vi "Wait For Single Object.vi"(8 "error in":errorcluster, 10 "Timeout":u32=4294967295 format="%d ms", 11 "Read Event in":refnum<class "Read Event.lvclass">) -> (0 "error out":errorcluster, 2 "Timed Out":bool, 3 "Read Event out":refnum<class "Read Event.lvclass">)   [LabVIEW 2019, in "PCANBasic.lvlib" / "Read Event.lvclass"]
doc: "Waits until the specified object is in the signaled state or the time-out interval elapses.\n\nThe time-out interval, in milliseconds. If a nonzero value is specified, the function waits until the object is signaled or the interval elapses. If dwMilliseconds is zero, the function does not enter a wait state if the object is not signaled; it always returns immediately. If dwMilliseconds is INFINITE (0xFFFFFFFF), the function will return only when the object is signaled."
uses:
  Read Event.lvclass
  Read Event.lvclass/Read Event.ctl
  PCANBasic.lvlib
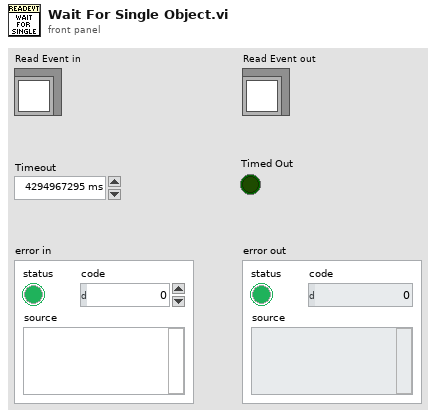
[diagram p1: front panel]
types:
  T1 = typedef "PCANBasic.lvlib/Read Event.lvclass/Event Handle.ctl" = u64
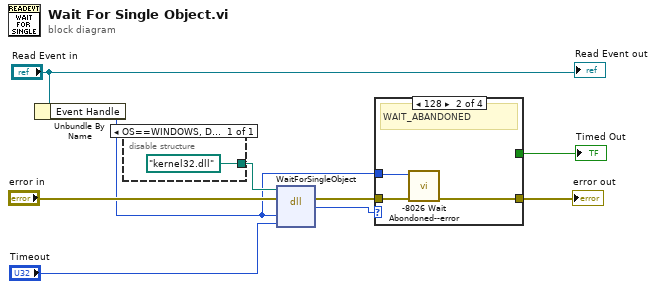
[diagram p0: block diagram]
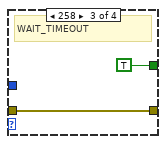
[diagram p3: hidden frame]
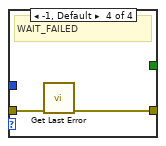
[diagram p4: hidden frame]
diagram:
  n1 = Unbundle By Name("Read Event in") -> ("Event Handle"=w2:T1)
  n2 = disable-structure shown="OS==WINDOWS, Default" {
    disable-tunnel: [path "kernel32.dll" ("path in")] -> w9
    frame condition #0 (active) {
    }
  }
  n3 = dll-call lib="?" fn="WaitForSingleObject"(path in=w9, error in="error in", "hdlEvent"=w2, "Timeout"="Timeout") -> (error out=w6:errorcluster, "result"=w5:u32)  [unwired: 3 in, 1 out]
  n4 = case "success?" shown="128" w5 {
    tunnel: w6 -> [w11 w14 w16 w18]
    tunnel: [w11 w13 w16 w17] -> w4
    tunnel: [_ _ TRUE _] -> w3
    tunnel: w2 -> [_ w12 _ _]
    frame 0 {
      # "WAIT_OBJECT_0"
    }
    frame 128 {
      # "WAIT_ABANDONED"
      n5 = call "-8026 Wait Abondoned--error.vi"("error in"=w14, "hdlEvent"=w12) -> ("error out"=w13:errorcluster)  [unwired: 8 in, 1 out]
    }
    frame 258 {
      # "WAIT_TIMEOUT"
    }
    frame -1, Default {
      # "WAIT_FAILED"
      n6 = call "Get Last Error.vi"("error in"=w18) -> ("error out"=w17:errorcluster)  [unwired: 10 in]
    }
  }
  "error out" <- w4
  "Timed Out" <- w3
  "Read Event out" <- "Read Event in"
